vi "TimeTrajectoryTest.vi"(8 "error in (no error)":errorcluster, 9 "Dest_array":T1(array[cluster]), 10 "TestParameters":T2, 11 "Game in":refnum<class "Game.lvclass">) -> (0 "error out":errorcluster, 2 "TestTeam out":refnum<class "Ally.lvclass">)   [LabVIEW 2023, in "Game.lvclass"]
uses:
  Game.lvclass
  Ally_class/Ally.lvclass
  C:/Users/ebert/Desktop/roboime/SSL_AI/Team_class/Team.lvclass
  Game.lvclass/Game.ctl
  Team_class/Team.lvclass/Team.ctl
  Navigation/Controls/typeOfUse.ctl
  Controls/Enviroment.ctl
  Object_class/Object.lvclass/Object.ctl
  Robot_class/Robot.lvclass/Robot.ctl
  <vilib>/Analysis/baseanly.llb/Unit Vector (DBL).vi
  <vilib>/Analysis/coordinate.llb/2D Cartesian Coordinate Rotation (Scalar).vi
  Robot_class/Read orientation.vi
  Object_class/Read position(x,y).vi
  Robot_class/Write v_tang.vi
  Robot_class/Write v_norm.vi
  Read TestTeam.vi
  Read AllyRef.vi
  Team_class/Read RobotRef.vi
  Team_class/Write RobotRef.vi
  Robot_class/Robot.lvclass
  C:/Users/ebert/Desktop/roboime/SSL_AI/Object_class/Object.lvclass
  Utilities_class/Utilities.lvclass
  <vilib>/Analysis/NI_AALPro.lvlib
  <vilib>/Analysis/NI_AALBase.lvlib
panel:
  in  "use model?":bool
  out "Distance":dbl
  out "Time remaining":dbl
  in  "Standard Trajectory":bool
  in  "time":dbl=0.5
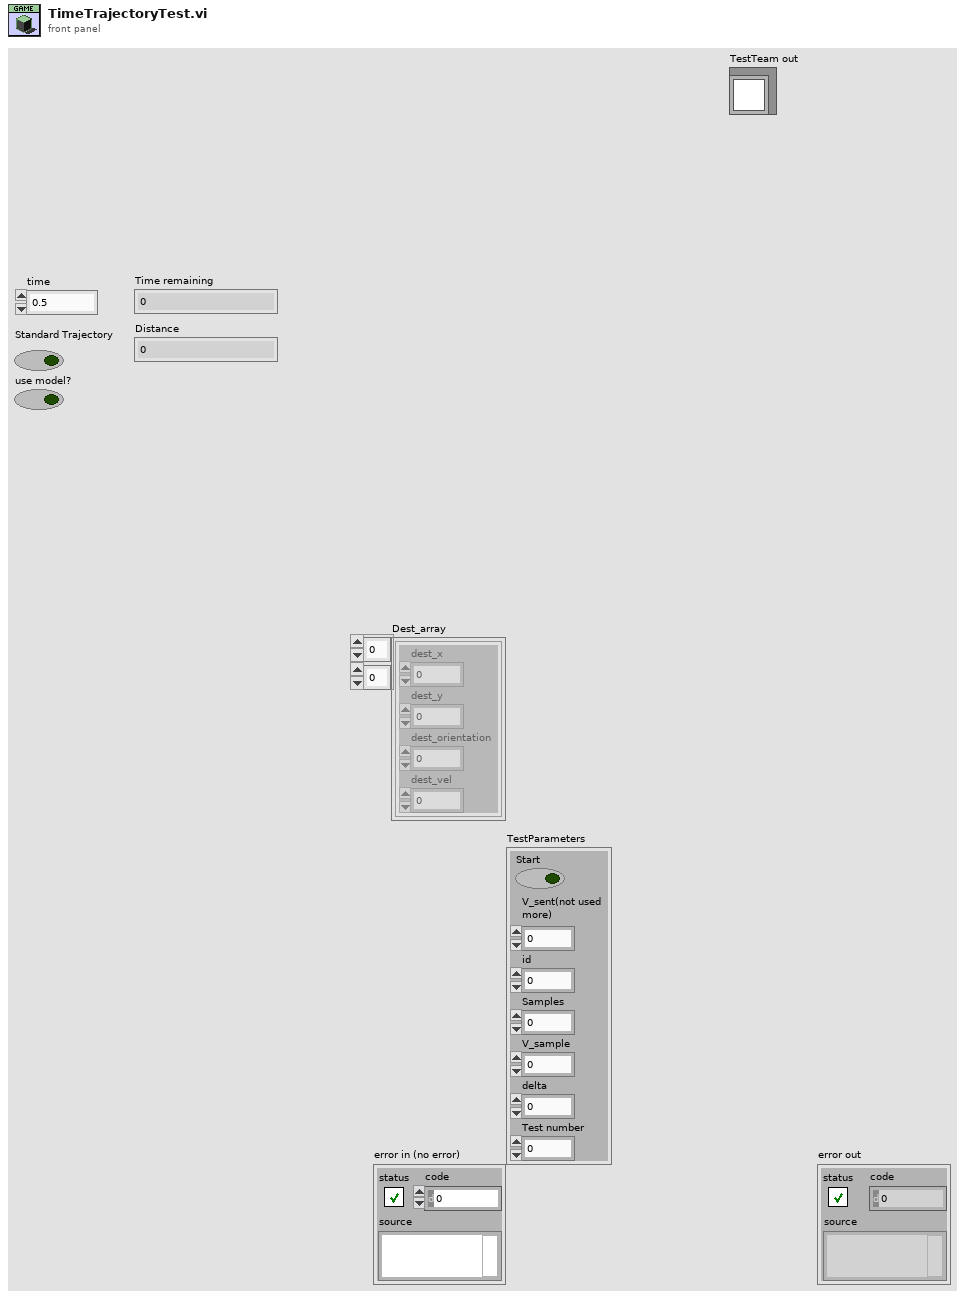
[diagram p1: front panel]
types:
  T1 = cluster{"dest_x":dbl, "dest_y":dbl, "dest_orientation":dbl, "dest_vel":dbl}[][]
  T2 = cluster{"Start":bool, "V_sent(not used\nmore)":dbl, "id":i32, "Samples":dbl, "V_sample":dbl, "delta":dbl, "Test number":dbl}
  T3 = typedef "typeOfUse.ctl" = enum16{"Navigation", "ZigZag", "grSimTest"}
  T4 = typedef "Enviroment.ctl" = enum16{"erForceSimulator", "grSim", "realGame"}
  T5 = cluster{"dest_x":dbl, "dest_y":dbl, "dest_orientation":dbl, "dest_vel":dbl}[]
  T6 = cluster{"dest_x":dbl, "dest_y":dbl, "dest_orientation":dbl, "dest_vel":dbl}
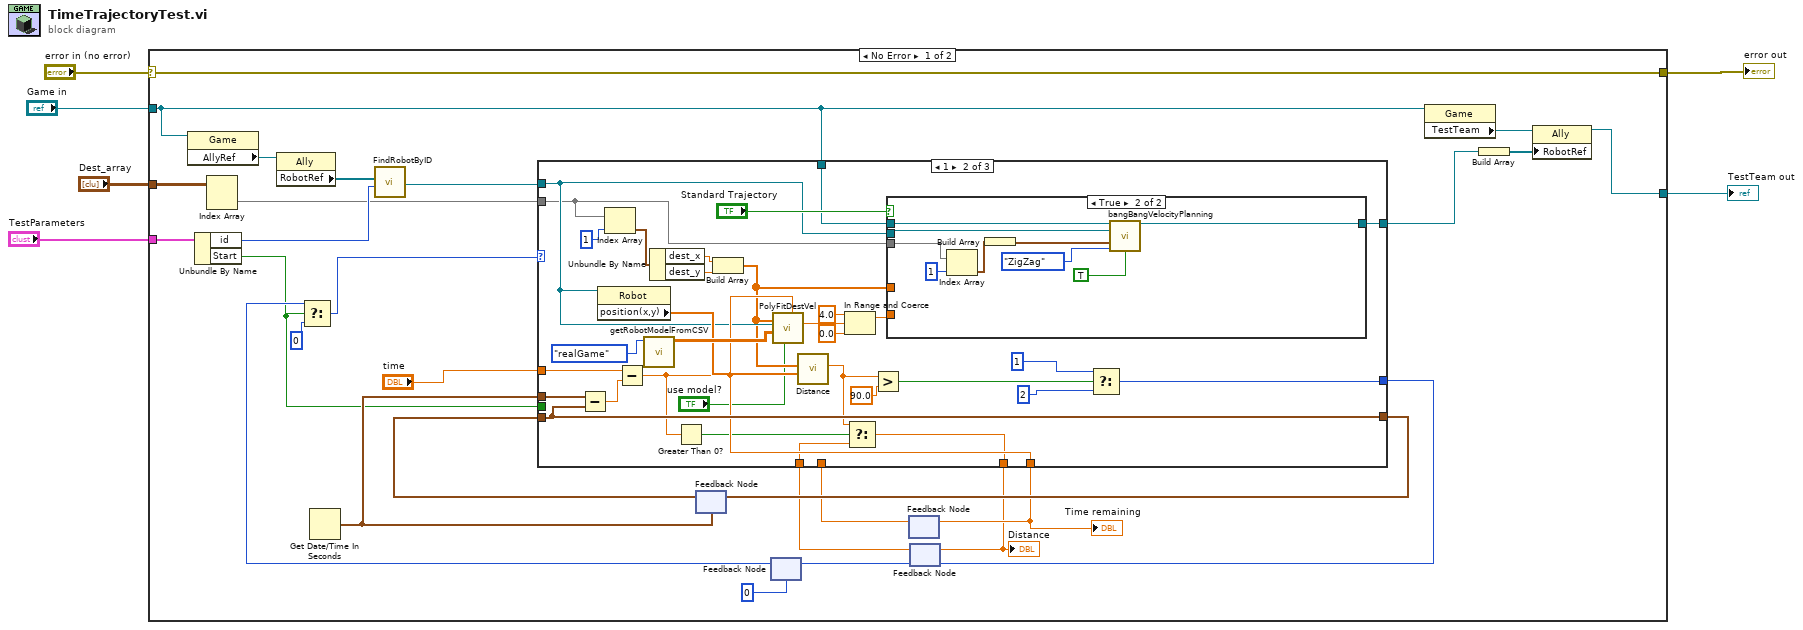
[diagram p0: block diagram]
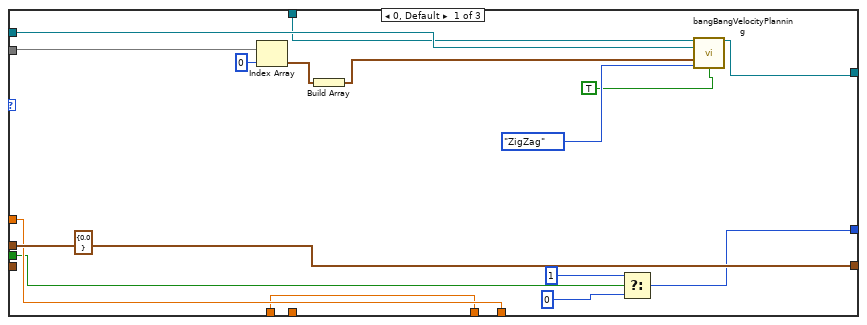
[diagram p2: hidden frame]
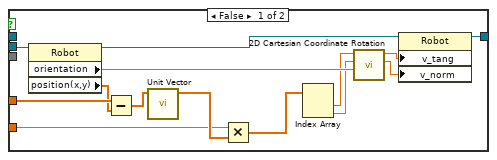
[diagram p3: hidden frame]
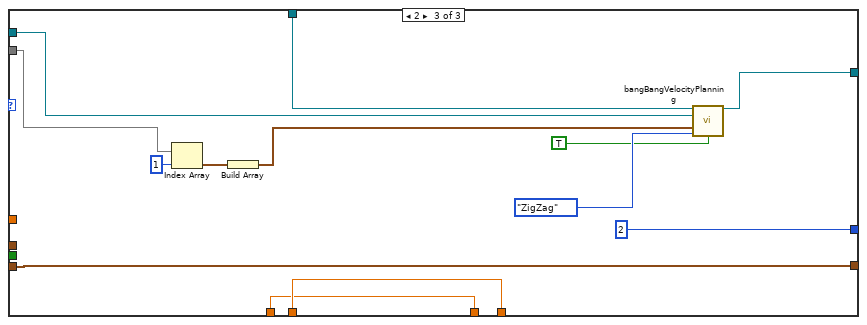
[diagram p4: hidden frame]
diagram:
  n1 = case shown="No Error" "error in (no error)" {
    selector: "error in (no error)" -> [w33 w118]
    tunnel: [w33 w118] -> w5
    tunnel: "Game in" -> [w8 _]
    tunnel: "TestParameters" -> [w30 _]
    tunnel: "Dest_array" -> [w28 _]
    tunnel: [w25 _] -> w1
    frame No Error {
      n2 = property class="Game"(reference=w8) -> ("AllyRef"=w32:refnum<class "Ally.lvclass">)  [unwired: 1 in, 2 out]
      n3 = Unbundle By Name(w30) -> ("id"=w29:i32, "Start"=w11:bool)
      n4 = Index Array(array=w28) -> (element=w20:T5)  [unwired: 2 in]
      n5 = property class="Ally"(reference=w32) -> ("RobotRef"=w31:refnum<class "Robot.lvclass">[])  [unwired: 1 in, 2 out]
      n6 = Get Date/Time In Seconds() -> (seconds since 1Jan1904=w22:timestamp)
      n7 = call "FindRobotByID.vi"("id"=w29, "RobotRef"=w31) -> ("Robot"=w19:refnum<class "Robot.lvclass">)  [unwired: 6 in, 3 out]
      n8 = feedback #1(w22) -> (w23:timestamp)
      n9 = feedback #2(0) -> (w14:i32)
      n10 = Select(t=w14, s=w11, f=0) -> (s? t:f=w12:i32)
      n11 = feedback #3() -> (w18:dbl)  [unwired: 1 in]
      n12 = feedback #4() -> (w10:dbl)  [unwired: 1 in]
      n13 = case shown="1" w12 {
        tunnel: w20 -> [w37 w50 w108]
        tunnel: w19 -> [w48 w57 w110]
        tunnel: [w49 w78 w117] -> w24
        tunnel: w23 -> [_ w78 w117]
        tunnel: w22 -> [w49 w79 _]
        tunnel: "time" -> [w47 w73 _]
        tunnel: w18 -> [_ _ w116]
        tunnel: [w47 w65 w116] -> w17
        tunnel: [w44 w66 2] -> w15
        tunnel: w11 -> [w46 _ _]
        tunnel: w10 -> [w42 w62 w114]
        tunnel: [w42 w61 w114] -> w9
        tunnel: w8 -> [w41 w58 w111]
        tunnel: [w38 w59 w109] -> w7
        frame 0, Default {
          (unwired) cluster{"dest_vel":dbl} {"dest_vel"=0.0} ("element")
          n14 = Index Array(array=w37, index=0) -> (element=w36:T6)
          n15 = Build Array(w36) -> (w34:T5)
          n16 = Select(t=1, s=w46, f=0) -> (s? t:f=w44:i32)
          n17 = call "bangBangVelocityPlanning.vi"("Game"=w41, "Robot in"=w48, "Dest_array"=w34, "type_of_use"=typeOfUse."ZigZag", "start"=TRUE) -> ("Robot out"=w38:refnum<class "Robot.lvclass">)  [unwired: 8 in, 2 out]
        }
        frame 1 {
          n18 = Subtract(x=w79, y=w78) -> (x-y=w72:dbl)
          n19 = property class="Robot"(reference=w57) -> ("position(x,y)"=w71:dbl[])  [unwired: 1 in, 2 out]
          n20 = Index Array(array=w50, index=1) -> (element=w77:T6)
          n21 = Subtract(x=w73, y=w72) -> (x-y=w65:dbl)
          n22 = call "getRobotModelFromCSV.vi"("Environment"=Enviroment."realGame") -> ("robotModel"=w74:dbl[][])  [unwired: 9 in, 1 out]
          n23 = Unbundle By Name(w77) -> ("dest_x"=w75:dbl, "dest_y"=w76:dbl)
          n24 = Greater Than 0?(x=w65) -> (x > 0?=w64:bool)
          n25 = Build Array(w75, w76) -> (w56:dbl[])
          n26 = call "PolyFitDestVel.vi"("TargetTime"=w65, "use model?"="use model?", "TargetPos"=w56, "robotModel"=w74, "Robot"=w57) -> ("vf"=w54:dbl)  [unwired: 4 in, 2 out]
          n27 = call "Distance.vi"("P1"=w71, "P2"=w56) -> ("Distance"=w63:dbl)  [unwired: 7 in, 2 out]
          n28 = In Range and Coerce(upper limit=4.0, x=w54, lower limit=0.0) -> (coerced(x)=w51:dbl)  [unwired: 1 out]
          n29 = Select(t=w63, s=w64, f=w62) -> (s? t:f=w61:dbl)
          n30 = Greater?(x=w63, y=90.0) -> (0:w69:bool)
          n31 = case shown="True" "Standard Trajectory" {
            tunnel: [w93 w102] -> w59
            tunnel: w58 -> [_ w101]
            tunnel: w57 -> [w95 w100]
            tunnel: w56 -> [w89 _]
            tunnel: w51 -> [w83 _]
            tunnel: w50 -> [_ w99]
            frame False {
              n32 = property class="Robot"(reference=w95) -> (reference out=w94:refnum<class "Robot.lvclass">, "orientation"=w90:dbl, "position(x,y)"=w88:dbl[])  [unwired: 1 in, 1 out]
              n33 = Subtract(x=w89, y=w88) -> (x-y=w85:dbl[])
              n34 = call-poly <vilib>:"Unit Vector.vi"("Input Vector"=w85) -> ("Unit Vector"=w84:dbl[])  [unwired: 8 in, 2 out]
              n35 = Multiply(x=w83, y=w84) -> (x*y=w82:dbl[])
              n36 = Index Array(array=w82) -> (element #1=w87:dbl, element #2=w86:dbl)  [unwired: 2 in]
              n37 = call-poly <vilib>:"2D Cartesian Coordinate Rotation.vi"("theta"=w90, "y"=w86, "x"=w87) -> ("y out"=w91:dbl, "x out"=w92:dbl)  [unwired: 6 in, 1 out]
              n38 = property class="Robot"(reference=w94, "v_tang"=w92, "v_norm"=w91) -> (reference out=w93:refnum<class "Robot.lvclass">)  [unwired: 1 in, 1 out]
            }
            frame True {
              n39 = Index Array(array=w99, index=1) -> (element=w97:T6)
              n40 = Build Array(w97) -> (w96:T5)
              n41 = call "bangBangVelocityPlanning.vi"("Game"=w101, "Robot in"=w100, "Dest_array"=w96, "type_of_use"=typeOfUse."ZigZag", "start"=TRUE) -> ("Robot out"=w102:refnum<class "Robot.lvclass">)  [unwired: 8 in, 2 out]
            }
          }
          n42 = Select(t=1, s=w69, f=2) -> (s? t:f=w66:i32)
        }
        frame 2 {
          n43 = Index Array(array=w108, index=1) -> (element=w106:T6)
          n44 = Build Array(w106) -> (w105:T5)
          n45 = call "bangBangVelocityPlanning.vi"("Game"=w111, "Robot in"=w110, "Dest_array"=w105, "type_of_use"=typeOfUse."ZigZag", "start"=TRUE) -> ("Robot out"=w109:refnum<class "Robot.lvclass">)  [unwired: 8 in, 2 out]
        }
      }
      "Time remaining" <- w17
      "Distance" <- w9
      n46 = feedback-in #1(w24) -> ()
      n47 = feedback-in #2(w15) -> ()
      n48 = feedback-in #3(w17) -> ()
      n49 = feedback-in #4(w9) -> ()
      n50 = property class="Game"(reference=w8) -> ("TestTeam"=w27:refnum<class "Ally.lvclass">)  [unwired: 1 in, 2 out]
      n51 = Build Array(w7) -> (w26:refnum<class "Robot.lvclass">[])
      n52 = property class="Ally"(reference=w27, "RobotRef"=w26) -> (reference out=w25:refnum<class "Ally.lvclass">)  [unwired: 1 in, 1 out]
    }
    frame Error {
    }
  }
  "error out" <- w5
  "TestTeam out" <- w1
